vi "Master_DAQ.vi"(8 "error in (no error)":errorcluster) -> (0 "error out":errorcluster)   [LabVIEW 2017]
doc: "Reads actual data from inputs or virtual data for testing. Converts the data into an array of double precision values and sends it to the user, HostMain.vi, and the main control loop."
uses:
  TypeDef_LoopPeriods.ctl
  Host/Libraries/TypeDef_NetworkStreamState.ctl
  Master_DataControl.ctl
  TypeDef_cRIOData.ctl
  IMU/TypeDef_IMUData.ctl
  CAN/TypeDef_BMSData.ctl
  CAN/TypeDef_BMS_Status.ctl
  CAN/MotorController/fixedMotorData.ctl
  CAN/MotorController/MotorStatus.ctl
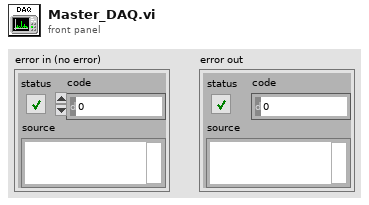
[diagram p1: front panel]
types:
  T1 = typedef "TypeDef_LoopPeriods.ctl" = cluster{"Control Period":i64, "DAQ Period":u32, "IMU Period":u32, "CAN Period":i64, "Nav Period":u32}
  T2 = typedef "TypeDef_NetworkStreamState.ctl" = enum16{"Wait", "Test", "Initialize", "Read/Write", "Terminate"}
  T3 = typedef "Master_DataControl.ctl" = cluster{"cRIO Data":T4, "IMU Data":T5, "BMS Data":T6, "Motor Data":T8}
  T4 = typedef "TypeDef_cRIOData.ctl" = cluster{"Time (ms)":dbl, "24V Battery (V)":dbl, "LowV Current (A)":dbl, "Fiducial Sensor (V)":dbl, "PV Pressure (psig)":dbl, "Flow Sensor (V)":dbl, "Temp Fairing (F)":dbl, "Temp Reservoir (F)":dbl, "HallEffect Right (in)":dbl, "HallEffect Left (in)":dbl, "PT Tank (psig)":dbl, "PT Clamp Right (psig)":dbl, "PT Clamp Left (psig)":dbl, "PT Brake (psig)":dbl, "PT Cooling (psig)":dbl, "Displacement (ft)":dbl, "Velocity (ft/s)":dbl}
  T5 = typedef "TypeDef_IMUData.ctl" = cluster{"x acceleration (g)":dbl, "Pressure (psia)":dbl, "Temperature (F)":dbl}
  T6 = typedef "TypeDef_BMSData.ctl" = cluster{"Max Cell Voltage (V)":dbl, "Max Cell ID":dbl, "Min Cell Voltage (V)":dbl, "Min Cell ID":dbl, "State of Charge (%)":dbl, "Average Voltage (V)":dbl, "Voltage Delta (V)":dbl, "Pack Current (A)":dbl, "Pack Voltage (V)":dbl, "Max Resistance (Ohm)":dbl, "Min Resistance (Ohm)":dbl, "Average Resistance (Ohm)":dbl, "Delta Resistance (Ohm)":dbl, "Highest Temperature(F)":dbl, "BmsStatus":T7}
  T7 = typedef "TypeDef_BMS_Status.ctl" = cluster{"isFault":bool, "isolationMonitoring":bool}
  T8 = typedef "fixedMotorData.ctl" = cluster{"Velo (RPM)":dbl, "MotorTemp(F)":dbl, "CtrlTemp(F)":dbl, "DcLinkVolt(V)":dbl, "ErrorCode":dbl, "motorStatus":T9, "isAlive":bool, "motorControllerState":u16}
  T9 = typedef "MotorStatus.ctl" = cluster{"isReady":bool, "isOn":bool, "isOperEn":bool, "isFault":bool, "isVoltEn":bool, "targetReached":bool, "isWarning":bool}
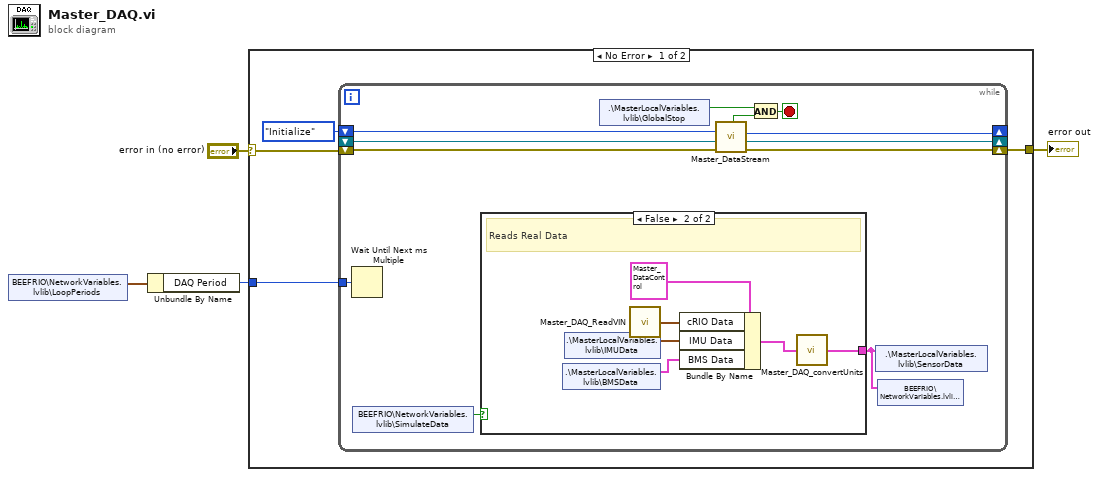
[diagram p0: block diagram]
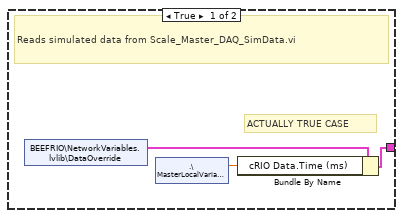
[diagram p2: hidden frame]
diagram:
  n1 = shared-variable "BEEFRIO\\NetworkVariables.lvlib\\LoopPeriods"() -> (w2:T1)  [unwired: 1 in, 1 out]
  n2 = Unbundle By Name(w2) -> ("DAQ Period"=w1:u32)
  n3 = case shown="No Error" "error in (no error)" {
    selector: "error in (no error)" -> [w8 w30]
    tunnel: [w7 w30] -> w3
    tunnel: w1 -> [w6 _]
    frame No Error {
      n4 = while {
        shift-right: [w13] -> w7
        shift-left: w8 -> [w15]
        shift-right: [w20] -> _
        shift-left: _ -> [w19]
        shift-right: [w18] -> _
        shift-left: TypeDef_NetworkStreamState."Initialize" ("Enum in") -> [w9]
        tunnel: w6 -> [w11]
        stop <- w17 stop-if-true
        n5 = Wait Until Next ms Multiple(millisecond multiple=w11) -> ()  [unwired: 1 out]
        n6 = shared-variable "BEEFRIO\\NetworkVariables.lvlib\\SimulateData"() -> (w12:bool)  [unwired: 1 in, 1 out]
        n7 = case shown="False" w12 {
          tunnel: [w23 w24] -> w10
          frame True {
            # "ACTUALLY TRUE CASE"
            # "Reads simulated data from Scale_Master_DAQ_SimData.vi"
            n8 = shared-variable "BEEFRIO\\NetworkVariables.lvlib\\DataOverride"() -> (w22:T3)  [unwired: 1 in, 1 out]
            n9 = shared-variable ".\\MasterLocalVariables.lvlib\\Time"() -> (w21:dbl)  [unwired: 1 in, 1 out]
            n10 = Bundle By Name(cluster=w22, "cRIO Data.Time (ms)"=w21) -> (w23:T3)
          }
          frame False {
            # "Reads Real Data"
            n11 = shared-variable ".\\MasterLocalVariables.lvlib\\BMSData"() -> (w26:T6)  [unwired: 1 in, 1 out]
            n12 = shared-variable ".\\MasterLocalVariables.lvlib\\IMUData"() -> (w27:T5)  [unwired: 1 in, 1 out]
            n13 = call "Master_DAQ_ReadVIN.vi"() -> ("cRIO Data"=w25:T4)  [unwired: 1 in]
            n14 = Bundle By Name(cluster=T3 {"cRIO Data"={"Time (ms)"=0.0, "24V Battery (V)"=0.0, "LowV Current (A)"=0.0, "Fiducial Sensor (V)"=0.0, "PV Pressure (psig)"=0.0, "Flow Sensor (V)"=0.0, "Temp Fairing (F)"=0.0, "Temp Reservoir (F)"=0.0, "HallEffect Right (in)"=0.0, "HallEffect Left (in)"=0.0, "PT Tank (psig)"=0.0, "PT Clamp Right (psig)"=0.0, "PT Clamp Left (psig)"=0.0, "PT Brake (psig)"=0.0, "PT Cooling (psig)"=0.0, "Displacement (ft)"=0.0, "Velocity (ft/s)"=0.0}, "IMU Data"={"x acceleration (g)"=0.0, "Pressure (psia)"=0.0, "Temperature (F)"=0.0}, "BMS Data"={"Max Cell Voltage (V)"=0.0, "Max Cell ID"=0.0, "Min Cell Voltage (V)"=0.0, "Min Cell ID"=0.0, "State of Charge (%)"=0.0, "Average Voltage (V)"=0.0, "Voltage Delta (V)"=0.0, "Pack Current (A)"=0.0, "Pack Voltage (V)"=0.0, "Max Resistance (Ohm)"=0.0, "Min Resistance (Ohm)"=0.0, "Average Resistance (Ohm)"=0.0, "Delta Resistance (Ohm)"=0.0, "Highest Temperature(F)"=0.0, "BmsStatus"={"isFault"=FALSE, "isolationMonitoring"=FALSE}}, "Motor Data"={"Velo (RPM)"=0.0, "MotorTemp(F)"=0.0, "CtrlTemp(F)"=0.0, "DcLinkVolt(V)"=0.0, "ErrorCode"=0.0, "motorStatus"={"isReady"=FALSE, "isOn"=FALSE, "isOperEn"=FALSE, "isFault"=FALSE, "isVoltEn"=FALSE, "targetReached"=FALSE, "isWarning"=FALSE}, "isAlive"=FALSE, "motorControllerState"=1}}, "cRIO Data"=w25, "IMU Data"=w27, "BMS Data"=w26) -> (w28:T3)
            n15 = call "Master_DAQ_convertUnits.vi"("Raw data in"=w28) -> ("Data out"=w24:T3)
          }
        }
        n16 = shared-variable ".\\MasterLocalVariables.lvlib\\GlobalStop"() -> (w14:bool)  [unwired: 1 in, 1 out]
        n17 = call "Master_DataStream.vi"("error in"=w15, "reader name in"=w19, "Enum in"=w9) -> ("error out"=w13:errorcluster, "reader name out"=w20:refnum<k21>, "Enum out"=w18:T2, "Boolean"=w16:bool)  [unwired: 5 in]
        n18 = And(x=w14, y=w16) -> (x .and. y?=w17:bool)
        n19 = shared-variable ".\\MasterLocalVariables.lvlib\\SensorData"(w10) -> ()  [unwired: 1 in, 1 out]
        n20 = shared-variable "BEEFRIO\\NetworkVariables.lvlib\\AllData"(w10) -> ()  [unwired: 1 in, 1 out]
      }
    }
    frame Error {
    }
  }
  "error out" <- w3
